vi "Global.vi"() -> ()   [LabVIEW 2014]
uses:
  Others (.ctl)/Control cluster.ctl
  <vilib>/LVH/AR Drone Toolkit/Decode NavData/Typedefs/NavData Demo.ctl
  <vilib>/LVH/AR Drone Toolkit/AR Drone.lvlib
panel:
  out "Control Cluster Out":T1={"Roll"=-0.03, "Pitch"=-0.052222222, "Vertical Speed"=0.0, "Yaw Speed"=0.0} {"Yaw Speed" scale=-1.0..1.0; "Vertical Speed" scale=-1.0..1.0; "Pitch" scale=-1.0..1.0; "Roll" scale=-1.0..1.0}
  out "Land/TakeOff":bool
  out "Rectangle":T2
  out "Gray IMAQ":T3(plugin-control)
  in  "stop":bool=TRUE
  out "Hover":bool
  out "NavData Out":T4
  out "Control Cluster":T1={"Roll"=-0.03, "Pitch"=-0.052222222, "Vertical Speed"=0.0, "Yaw Speed"=0.0} {"Yaw Speed" scale=-1.0..1.0; "Vertical Speed" scale=-1.0..1.0; "Pitch" scale=-1.0..1.0; "Roll" scale=-1.0..1.0}
  out "B&W IMAQ with rectangle":T3(plugin-control)
  out "Raw video":picture
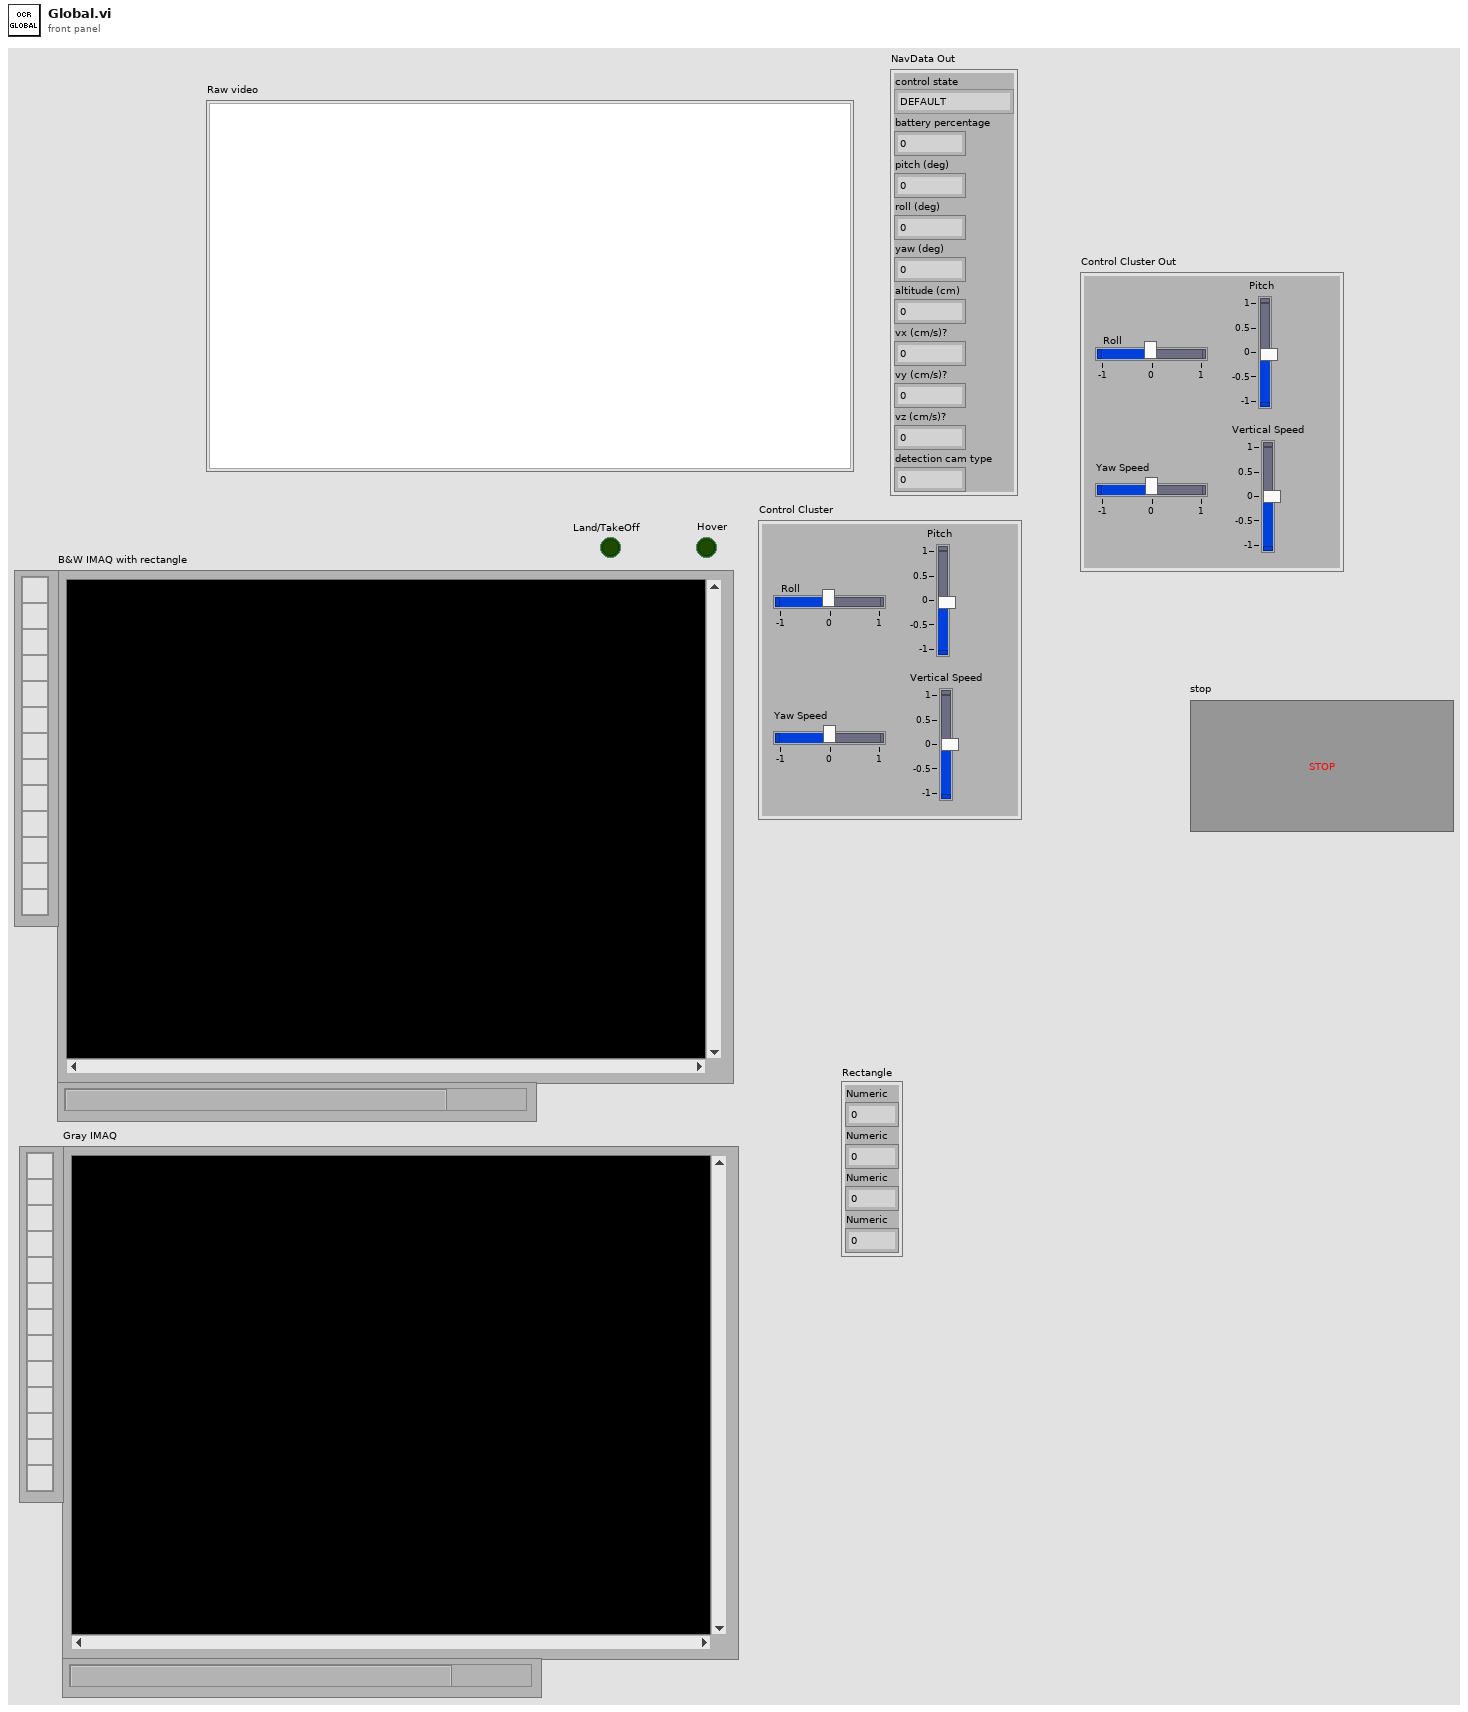
[diagram p1: front panel]
types:
  T1 = typedef "Control cluster.ctl" = cluster{"Roll":sgl, "Pitch":sgl, "Vertical Speed":sgl, "Yaw Speed":sgl}
  T2 = cluster{"Numeric":dbl, "Numeric":dbl, "Numeric":dbl, "Numeric":dbl}
  T3 = typedef "IMAQ Image.ctl" = refnum<image>
  T4 = typedef "AR Drone.lvlib/NavData Demo.ctl" = cluster{"control state":enum32{"DEFAULT", "INIT", "LANDING", "FLYING", "HOVERING", "TEST", "TRANS_TAKEOFF", "TRANS_GOTOFIX", "TRANS_LANDING"}, "battery percentage":u32, "pitch (deg)":sgl, "roll (deg)":sgl, "yaw (deg)":sgl, "altitude (cm)":u32, "vx (cm/s)?":sgl, "vy (cm/s)?":sgl, "vz (cm/s)?":sgl, "detection cam type":u32}
diagram:
